vi "Channel_WriteLog.vi"(0 "Channel in":refnum<class "Channel.lvclass">, 1 "tdms file":refnum<k34>, 2 "Loop Counter":i32, 5 "Group Name":string, 7 "t0":timestamp, 9 "dt per loop":dbl, 11 "error in (no error)":errorcluster) -> (4 "Channel out":refnum<class "Channel.lvclass">, 6 "tdms file out":refnum<k34>, 15 "error out":errorcluster)   [LabVIEW 2023, in "Channel.lvclass"]
doc: "Write channel to file - is a top level VI to diceminate whether to call the corresponding waveform or standard channel write method."
uses:
  Channel.lvclass
  Channel.lvclass/Channel.ctl
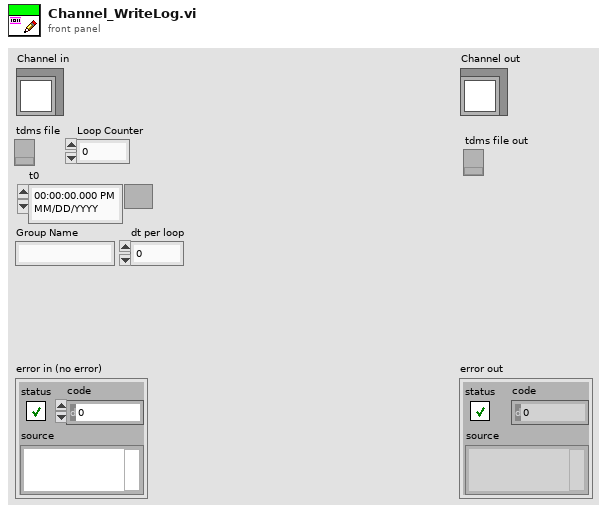
[diagram p1: front panel]
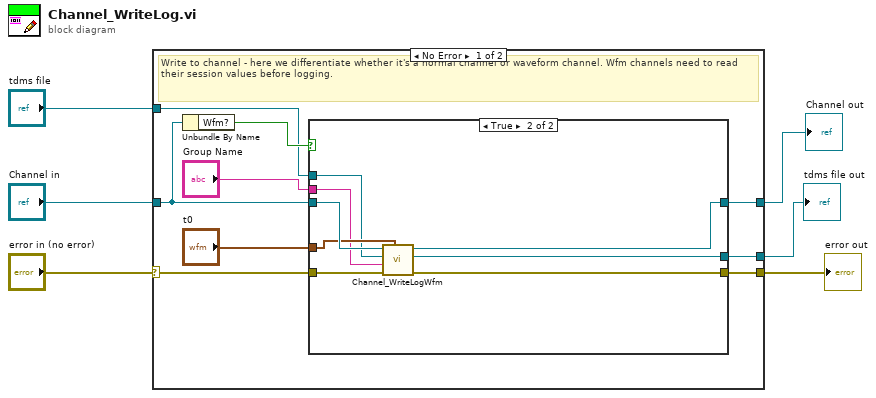
[diagram p0: block diagram]
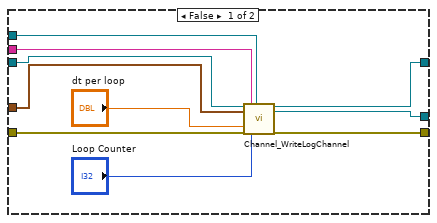
[diagram p2: hidden frame]
diagram:
  n1 = case shown="No Error" "error in (no error)" {
    selector: "error in (no error)" -> [w15 w36]
    tunnel: [w14 w36] -> w5
    tunnel: [w11 w35] -> w3
    tunnel: "Channel in" -> [w12 w35]
    tunnel: [w8 w34] -> w2
    tunnel: "tdms file" -> [w7 w34]
    frame No Error {
      # "Write to channel - here we differentiate whether it's a normal channel or waveform channel. Wfm channels need to read their session values before logging."
      n2 = Unbundle By Name(w12) -> ("Wfm?"=w13:bool)
      n3 = case shown="True" w13 {
        tunnel: w15 -> [w25 w33]
        tunnel: [w24 w32] -> w14
        tunnel: w12 -> [w23 w31]
        tunnel: [w22 w30] -> w11
        tunnel: "t0" -> [w19 w29]
        tunnel: w7 -> [w20 w28]
        tunnel: "Group Name" -> [w21 w27]
        tunnel: [w16 w26] -> w8
        frame False {
          n4 = call-dynamic "Channel_WriteLogChannel.vi"("Channel in"=w23, "Time"=w19, "dt per loop"="dt per loop", "error in (no error)"=w25, "Group Name"=w21, "Loop Counter"="Loop Counter", "tdms file"=w20) -> ("Channel out"=w22:refnum<class "Channel.lvclass">, "tdms file out"=w16:refnum<k34>, "error out"=w24:errorcluster)  [unwired: 10 in]
        }
        frame True {
          n5 = call-dynamic "Channel_WriteLogWfm.vi"("t0"=w29, "error in (no error)"=w33, "Group Name"=w27, "tdms file"=w28, "Channel in"=w31) -> ("error out"=w32:errorcluster, "tdms file out"=w26:refnum<k34>, "Channel out"=w30:refnum<class "Channel.lvclass">)  [unwired: 4 in]
        }
      }
    }
    frame Error {
    }
  }
  "error out" <- w5
  "Channel out" <- w3
  "tdms file out" <- w2
